vi "Configure Segment Start Stop.vi"(6 "Stop Freq (1E+6 Hz)":dbl=1000000.0, 7 "Start Freq (1E+6 Hz)":dbl=1000000.0, 8 "error in (no error)":errorcluster, 9 "Segment Number (1)":i32=1, 10 "Channel (1)":i32=1, 11 "VISA resource name":refnum<visa-resource-name>) -> (0 "error out":errorcluster, 3 "VISA resource name out":refnum<visa-resource-name>)   [LabVIEW 2018, in "Keysight PNA Series.lvlib"]
doc: "Sets the Start and Stop Frequency for the specified sweep segment."
uses:
  Keysight PNA Series.lvlib
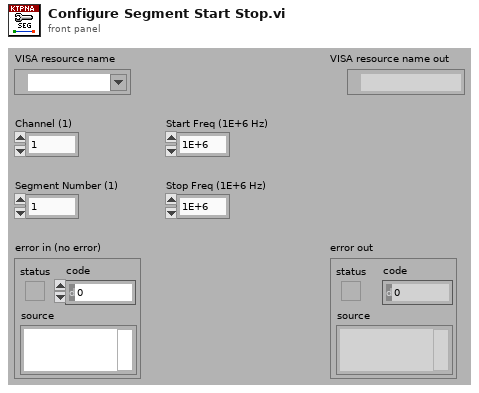
[diagram p1: front panel]
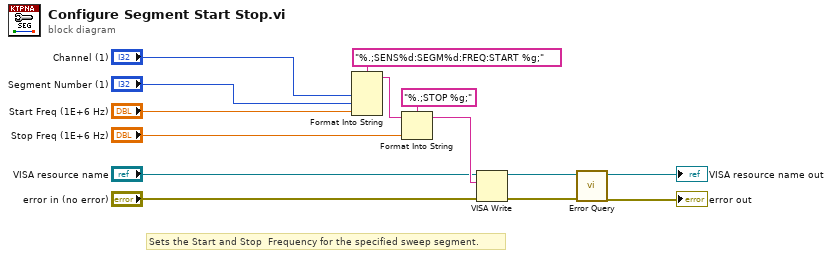
[diagram p0: block diagram]
diagram:
  # "Sets the Start and Stop  Frequency for the specified sweep segment."
  n1 = Format Into String(format string="%.;SENS%d:SEGM%d:FREQ:START %g;", "Channel (1)", "Segment Number (1)", "Start Freq (1E+6 Hz)") -> (resulting string=w10:string)  [unwired: 2 in, 1 out]
  n2 = Format Into String(format string="%.;STOP %g;", initial string=w10, "Stop Freq (1E+6 Hz)") -> (resulting string=w8:string)  [unwired: 1 in, 1 out]
  n3 = VISA Write(VISA resource name="VISA resource name", write buffer=w8, error in (no error)="error in (no error)") -> (VISA resource name out=w5:refnum<visa-resource-name>, error out=w4:errorcluster)  [unwired: 1 out]
  n4 = call "Error Query.vi"("error in (no error)"=w4, "VISA resource name"=w5) -> ("error out"=→"error out":errorcluster, "VISA resource name out"=→"VISA resource name out":refnum<visa-resource-name>)  [unwired: 6 in, 2 out]
